vi "Open.vi"(8 "Error In":errorcluster, 10 "Mode":T1, 11 "EZ430-Chronos Config":T3) -> (0 "Error Out":errorcluster, 3 "EZ430-Chronos Ref":T2)   [LabVIEW 2011, in "LVH-EZ430.lvlib"]
doc: "Open a connection to the EZ430-Chronos."
uses:
  LVH-EZ430.lvlib
  Private/Type Defs/EZ430-Chronos Config.ctl
  Private/Type Defs/EZ430-Chronos Ref.ctl
  Private/Type Defs/Mode.ctl
  <vilib>/Instr/_visa.llb/VISA Configure Serial Port (Instr).vi
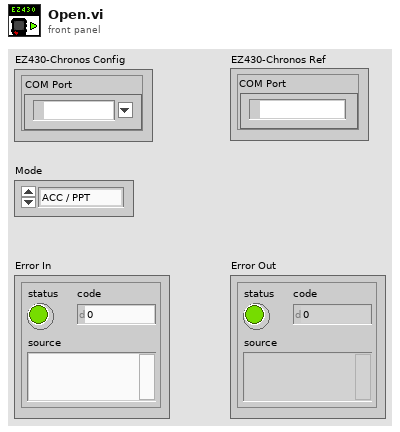
[diagram p1: front panel]
types:
  T1 = typedef "LVH-EZ430.lvlib/Mode.ctl" = enum16{"ACC / PPT"}
  T2 = typedef "LVH-EZ430.lvlib/EZ430-Chronos Ref.ctl" = cluster{"COM Port":refnum<visa-resource-name>}
  T3 = typedef "LVH-EZ430.lvlib/EZ430-Chronos Config.ctl" = cluster{"COM Port":refnum<visa-resource-name>}
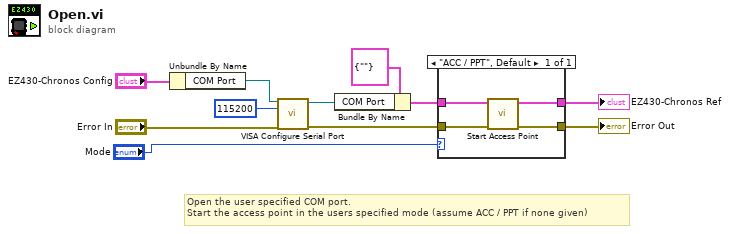
[diagram p0: block diagram]
diagram:
  # "Open the user specified COM port.\nStart the access point in the users specified mode (assume ACC / PPT if none given)"
  n1 = Unbundle By Name("EZ430-Chronos Config") -> ("COM Port"=w10:refnum<visa-resource-name>)
  n2 = call-poly "VISA Configure Serial Port"("VISA resource name"=w10, "baud rate (9600)"=u32 115200, "error in (no error)"="Error In") -> ("VISA resource name out"=w6:refnum<visa-resource-name>, "error out"=w3:errorcluster)  [unwired: 11 in]
  n3 = Bundle By Name(cluster=T2 {"COM Port"=""} ("EZ430-Chronos Config"), "COM Port"=w6) -> (w5:T2)
  n4 = case shown="\"ACC / PPT\", Default" "Mode" {
    tunnel: w5 -> [w15]
    tunnel: [w14] -> w4
    tunnel: w3 -> [w13]
    tunnel: [w12] -> w1
    frame "ACC / PPT", Default {
      n5 = call "Start Access Point.vi"("Error In"=w13, "EZ430-Chronos Ref"=w15) -> ("Error Out"=w12:errorcluster, "EZ430-Chronos Ref"=w14:T2)  [unwired: 8 in]
    }
  }
  "Error Out" <- w1
  "EZ430-Chronos Ref" <- w4
